vi "Temperature Warnings.vi"(0 "현재 온도":dbl, 11 "에러 입력":cluster{"상태":bool, "코드":i32, "소스":string}) -> ()   [LabVIEW 2018]
doc: "이 VI는 현재 온도 및 리미트 셋팅에 기반하여 기상 관측기에 출력할 문자열을 결정하는데 사용됩니다.\n\n입력: 현재 온도(DBL), 최저 온도(DBL) 및 최고 온도(DBL).\n출력: 경고 텍스트(문자열) 및 경고?(불리언)."
panel:
  out "에러 출력":cluster{"상태":bool, "코드":i32, "소스":string}
  out "경고 텍스트":string="경고 없음"
  out "경고?":bool
  in  "최저 온도":dbl
  in  "최고 온도":dbl
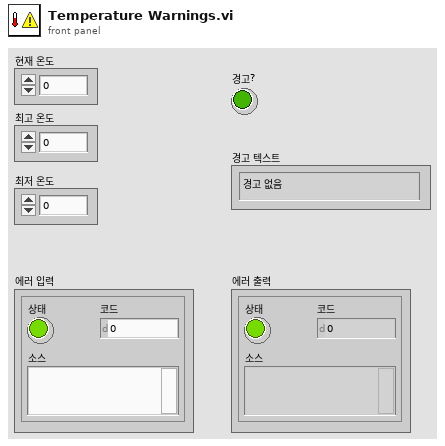
[diagram p1: front panel]
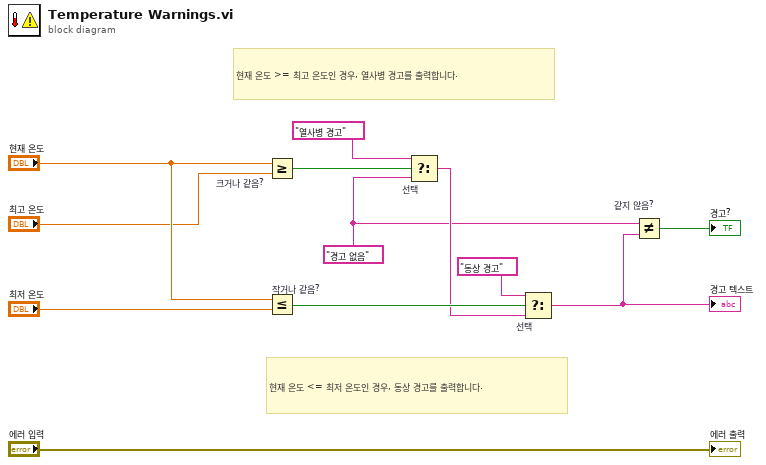
[diagram p0: block diagram]
diagram:
  w2 = "경고 없음" ("f")
  # "현재 온도 >= 최고 온도인 경우, 열사병 경고를 출력합니다."
  # "현재 온도 <= 최저 온도인 경우, 동상 경고를 출력합니다."
  n1 = Greater Or Equal? "크거나 같음?"(x="현재 온도", y="최고 온도") -> (x >= y?=w7:bool)
  n2 = Less Or Equal? "작거나 같음?"(x="현재 온도", y="최저 온도") -> (x <= y?=w4:bool)
  n3 = Select "선택"(t="열사병 경고", s=w7, f=w2) -> (s? t:f=w3:string)
  n4 = Select "선택"(t="동상 경고", s=w4, f=w3) -> (s? t:f=w8:string)
  "경고 텍스트" <- w8
  n5 = Not Equal? "같지 않음?"(x=w2, y=w8) -> (x != y?=→"경고?":bool)
  "에러 출력" <- "에러 입력"
